vi "Read Panel.vi"(8 "error in (no error)":errorcluster, 11 "Panel Actor Form Config in":refnum<class "Panel Actor Form Config.lvclass">) -> (0 "error out":errorcluster, 2 "Panel.lvlib:Panel.lvclass":refnum<class "Panel.lvclass">, 3 "Panel Actor Form Config out":refnum<class "Panel Actor Form Config.lvclass">)   [LabVIEW 2020, in "Panel Actor Form Config.lvclass"]
uses:
  Panel Actor Form Config.lvclass
  <vilib>/MGI/Panel Manager/Panel/Panel/Panel.lvclass
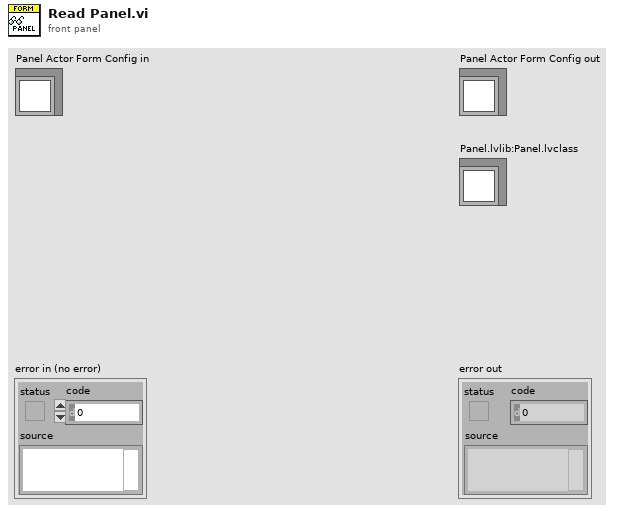
[diagram p1: front panel]
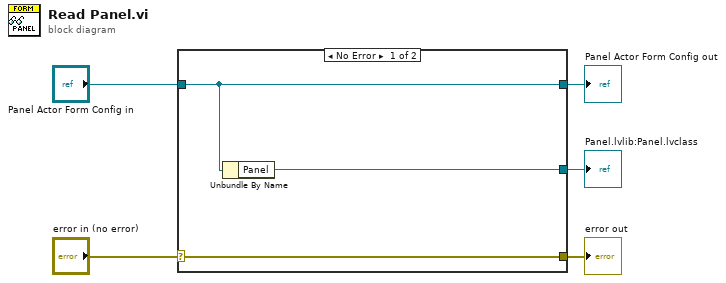
[diagram p0: block diagram]
diagram:
  n1 = case shown="No Error" "error in (no error)" {
    selector: "error in (no error)" -> [w8 w9]
    tunnel: [w8 w9] -> w4
    tunnel: [w7 w10] -> w2
    tunnel: "Panel Actor Form Config in" -> [w7 w10]
    tunnel: [w6 _] -> w1
    frame No Error {
      n2 = Unbundle By Name(w7) -> ("Panel"=w6:refnum<class "Panel.lvclass">)
    }
    frame Error {
    }
  }
  "error out" <- w4
  "Panel Actor Form Config out" <- w2
  "Panel.lvlib:Panel.lvclass" <- w1
